vi "YokogawaGS200SweepAlexei.vi"() -> ()   [LabVIEW 2019]
panel:
  in  "INFINITE RUN status":bool caption="INFINITE RUN"
  in  "Set Time (s)":dbl=1.0 min=0.1 max=100.0 format="%.3f"
  out "Output Volt":dbl min=-10.0 max=10.0 format="%^.3e"
  in  "INFINITE RUN":bool
  in  "MODE:":enum32{"RAMP", "TRIANGLE"}(radio)=enum."TRIANGLE"
  in  "Step |Volt| (abs. value)":dbl=0.05 min=-1.0 max=1.0 format="%^.3e"
  in  "Delay per step OR ramp (s)":dbl=1.0 min=0.1 max=100.0 format="%.3f"
  in  "pause sweep":bool
  in  "Compliance Current":dbl format="%.3f"
  in  "Stop Volt":dbl=1.0 min=-10.0 max=10.0 format="%^.3e"
  in  "Start Volt":dbl min=-10.0 max=10.0 format="%^.3e"
  in  "Output Off":bool
  in  "Start Sweep":bool
  in  "Setup":bool
  in  "VISA resource name":refnum<visa-resource-name>
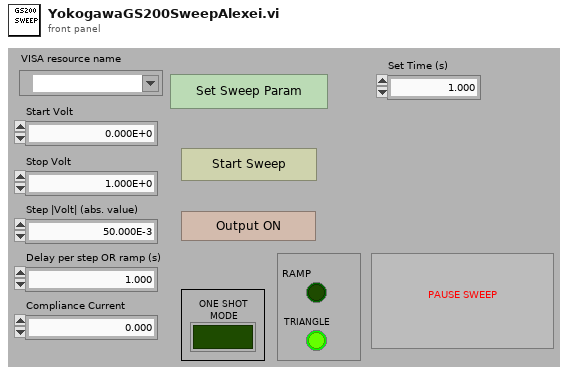
[diagram p1: front panel]
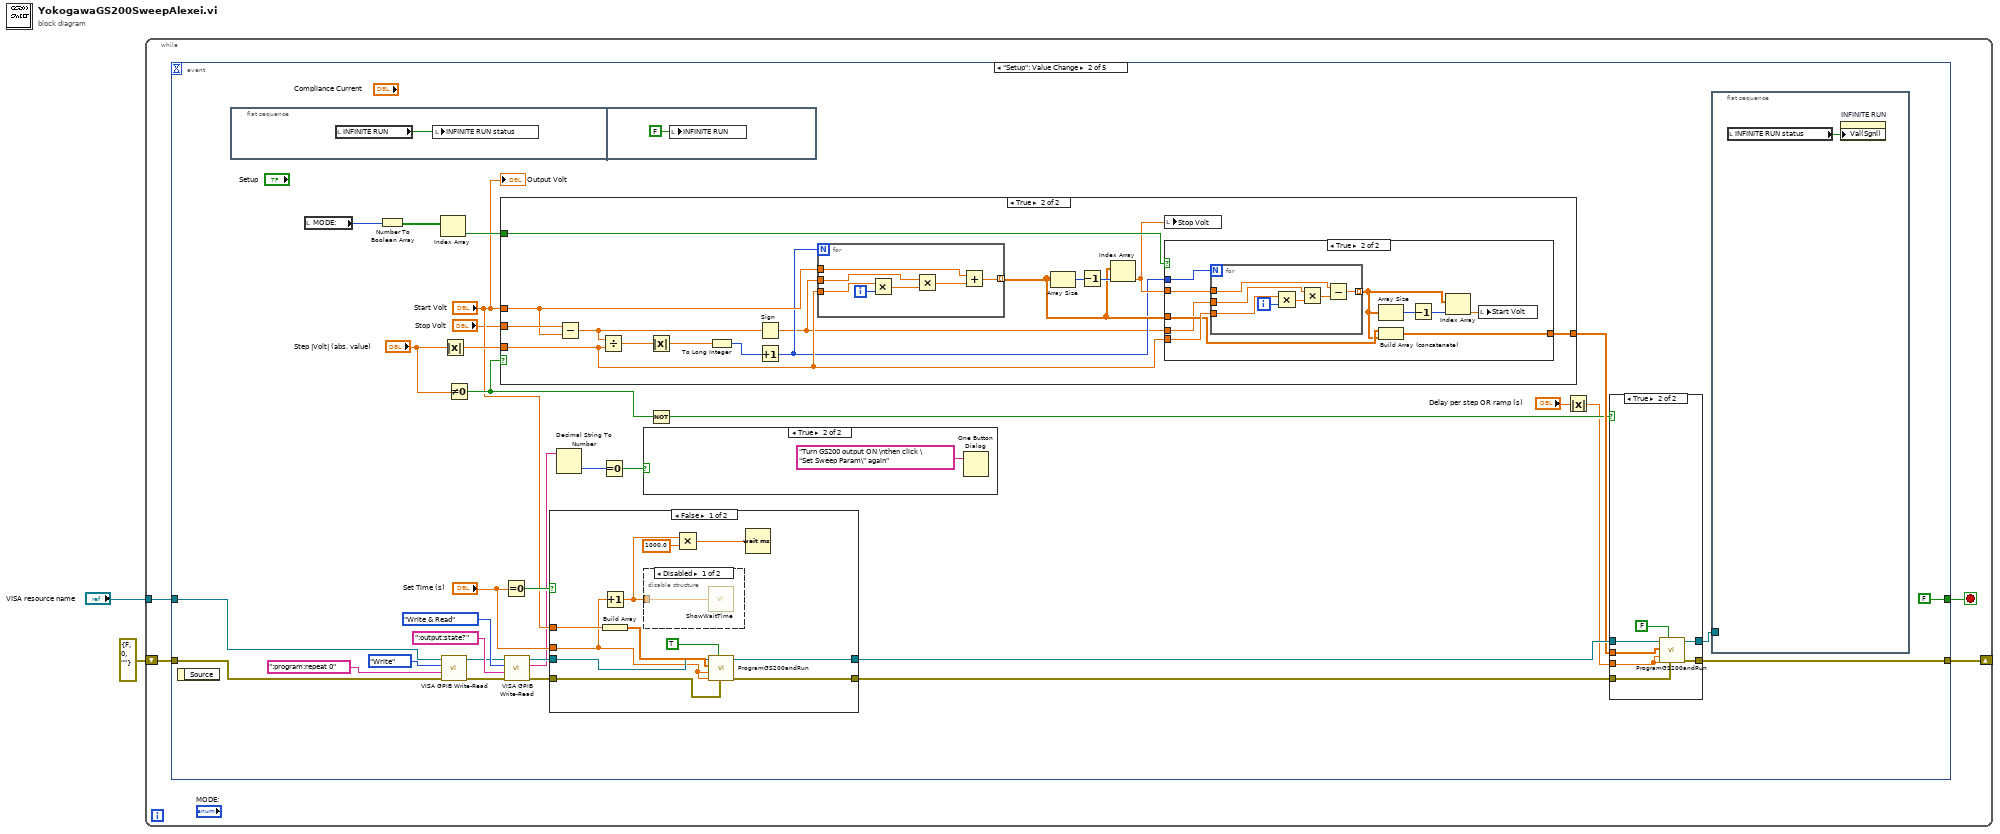
[diagram p0: block diagram]
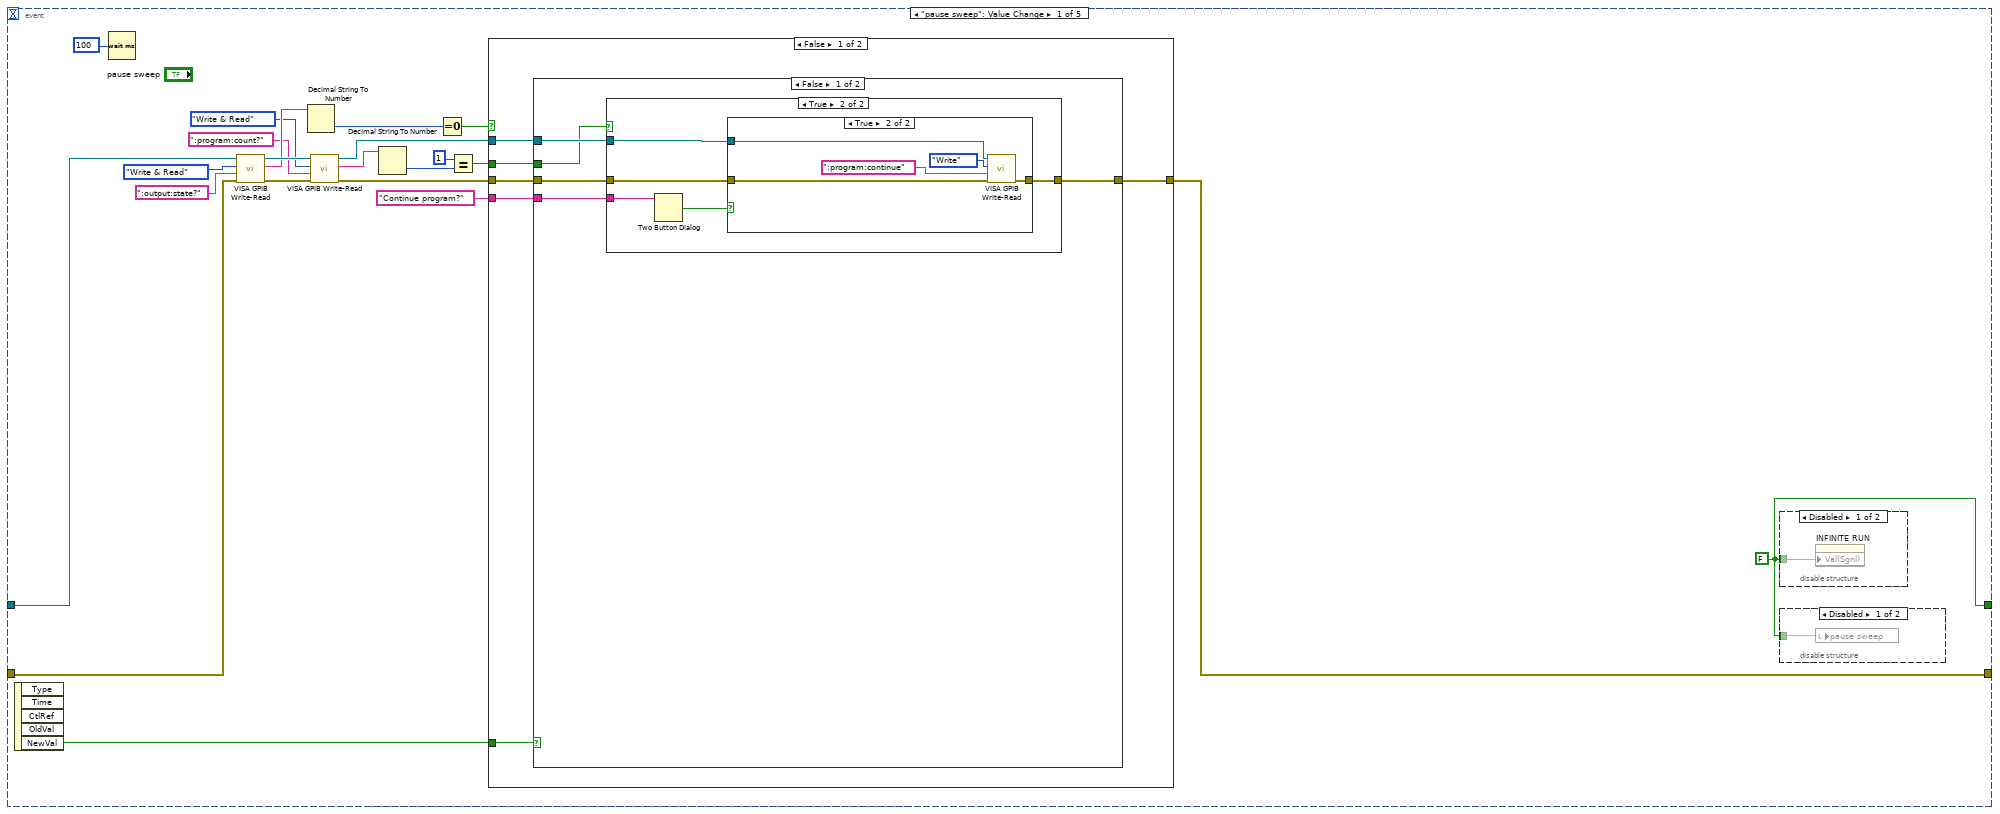
[diagram p2: hidden frame]
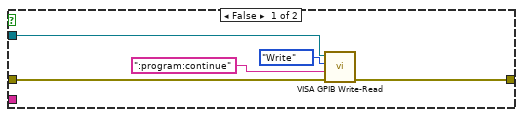
[diagram p4: hidden frame]
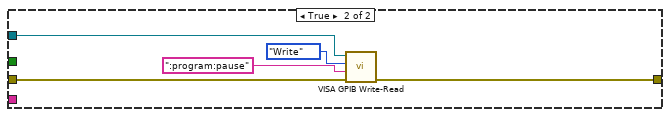
[diagram p6: hidden frame]
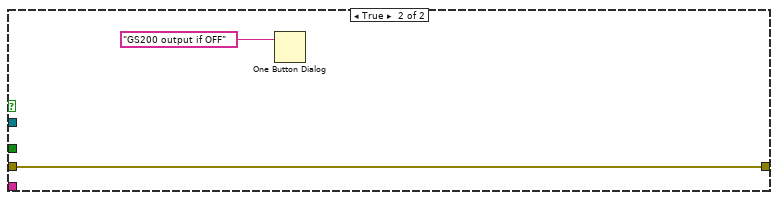
[diagram p7: hidden frame]
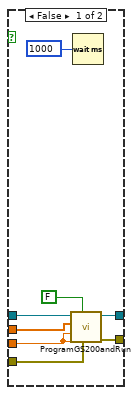
[diagram p9: hidden frame]
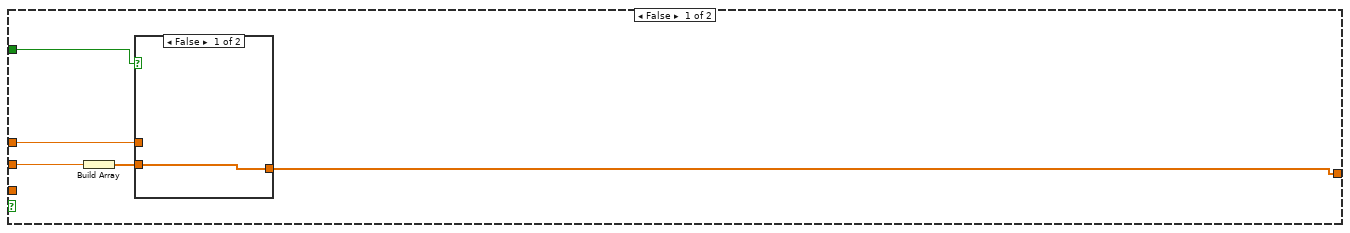
[diagram p11: hidden frame]
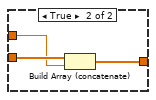
[diagram p12: hidden frame]
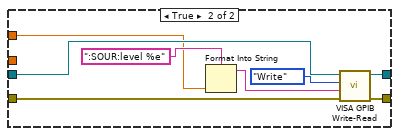
[diagram p15: hidden frame]
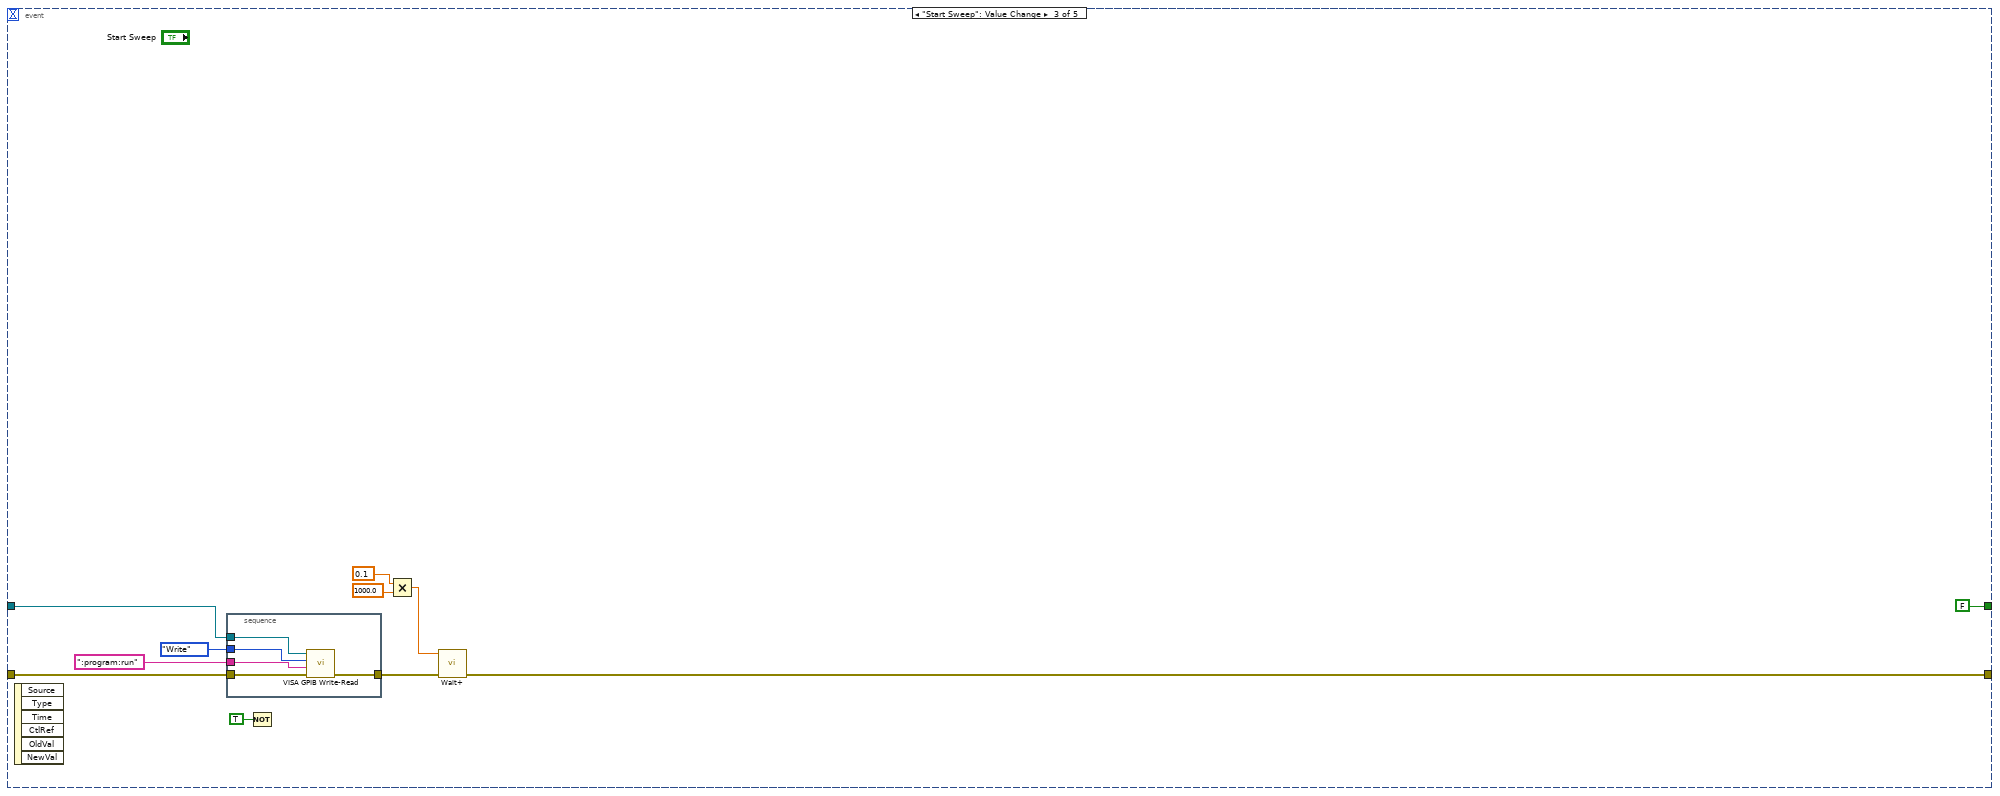
[diagram p16: hidden frame]
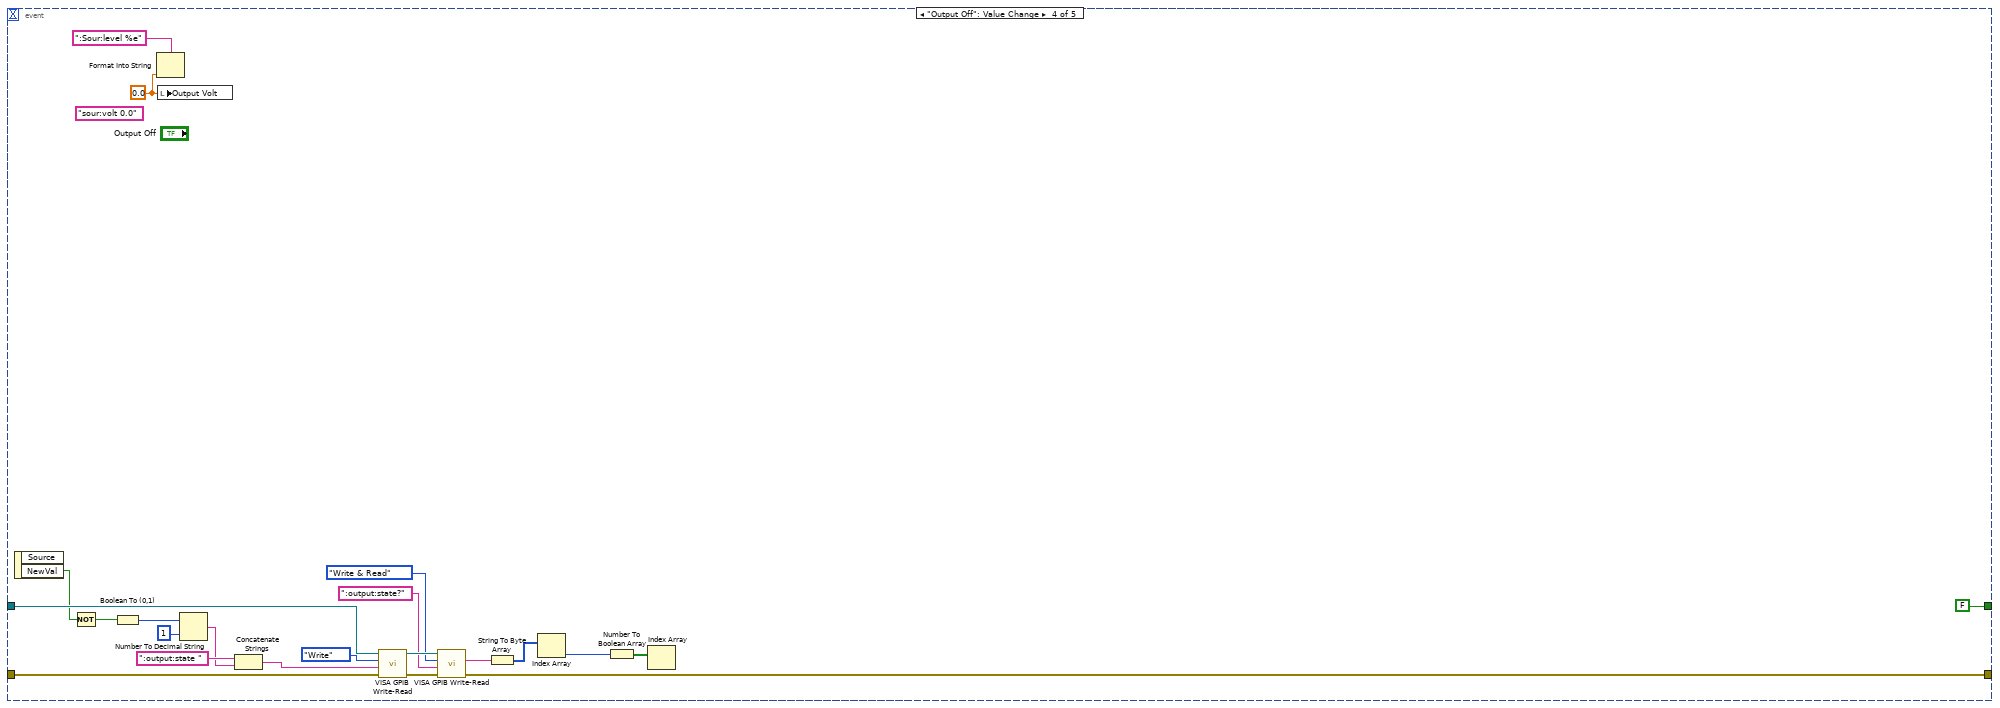
[diagram p17: hidden frame]
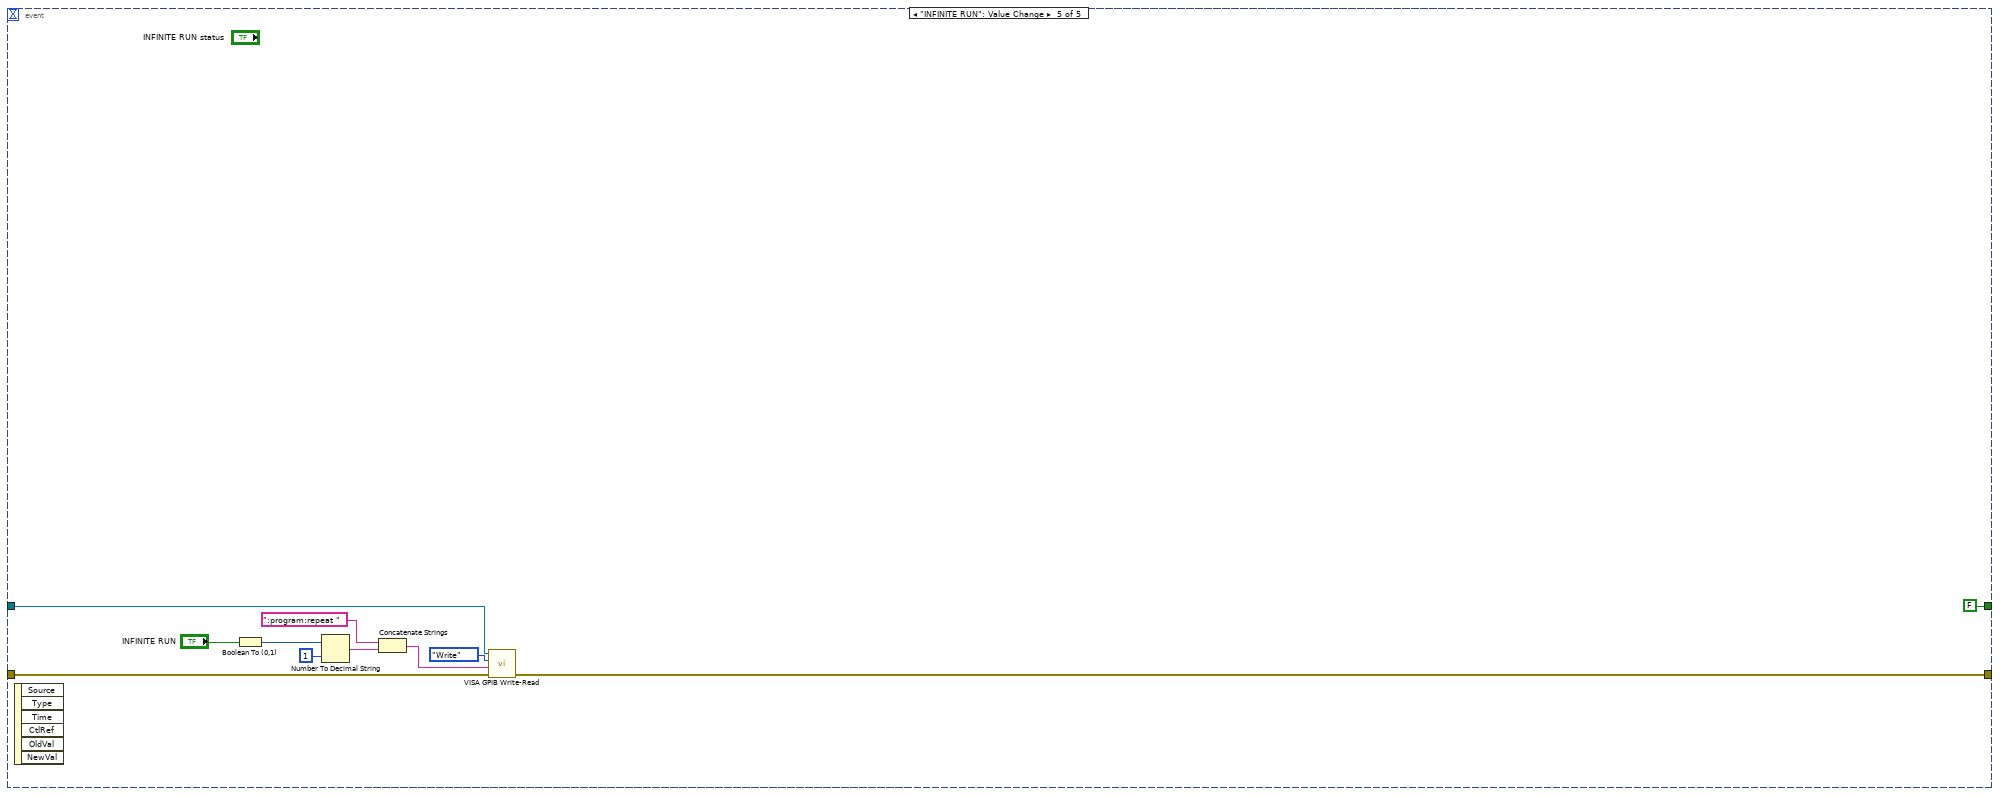
[diagram p18: hidden frame]
diagram:
  n1 = while {
    shift-right: [w5] -> _
    shift-left: errorcluster {"status"=FALSE, "code"=0, "source"=""} ("error out") -> [w4]
    tunnel: "VISA resource name" -> [w3]
    stop <- w6 stop-if-true
    n2 = event shown="[1] \"Setup\": Value Change" {
      selector: _ -> [_ _ _ _ _]
      dyn-events: _ -> [_ _ _ _ _]
      timeout: _ -> [_ _ _ _ _]
      tunnel: w3 -> [w26 w79 w195 w221 w227]
      tunnel: [w28 FALSE ("NewVal") FALSE ("NewVal") FALSE ("NewVal") FALSE ("NewVal")] -> w6
      tunnel: [w7 w67 w193 w220 w224] -> w5
      tunnel: w4 -> [w8 w66 w194 w219 w225]
      event "pause sweep": Value Change {
        w28 = FALSE ("stop")
        n3 = event-data() -> ("NewVal"=w27:bool)  [unwired: 1 in, 4 out]
        n4 = Wait (ms)(milliseconds to wait=u32 100) -> ()  [unwired: 1 out]
        n5 = call "VISA GPIB Write-Read.vi"("error in (no error)"=w8, "Command"=":output:state?" ("String to Write"), "Action"=enum16{"Write", "Read", "Write & Read"}."Write & Read", "VISA resource name"=w26) -> ("error out"=w10:errorcluster, "String Returned"=w19:string, "dup VISA Session"=w25:refnum<visa-resource-name>)  [unwired: 4 in, 1 out]
        n6 = Decimal String To Number(string=w19) -> (number=w20:i32)  [unwired: 2 in, 1 out]
        n7 = call "VISA GPIB Write-Read.vi"("error in (no error)"=w10, "Command"=":program:count?" ("String to Write"), "Action"=enum16{"Write", "Read", "Write & Read"}."Write & Read", "VISA resource name"=w25) -> ("error out"=w9:errorcluster, "String Returned"=w15:string, "dup VISA Session"=w16:refnum<visa-resource-name>)  [unwired: 4 in, 1 out]
        n8 = Decimal String To Number(string=w15) -> (number=w14:i32)  [unwired: 2 in, 1 out]
        n9 = Equal To 0?(x=w20) -> (x = 0?=w24:bool)
        n10 = Equal?(x=1, y=w14) -> (x = y?=w12:bool)
        n11 = case shown="False" w24 {
          tunnel: w16 -> [w35 _]
          tunnel: w27 -> [w34 _]
          tunnel: w12 -> [w33 _]
          tunnel: "Continue program?" ("message") -> [w32 _]
          tunnel: w9 -> [w31 w62]
          tunnel: [w30 w62] -> w7
          frame False {
            n12 = case shown="False" w34 {
              tunnel: w35 -> [w40 w59]
              tunnel: w33 -> [w39 _]
              tunnel: w32 -> [w38 _]
              tunnel: w31 -> [w37 w57]
              tunnel: [w36 w58] -> w30
              frame False {
                n13 = case shown="True" w39 {
                  tunnel: w40 -> [w43 w50]
                  tunnel: w38 -> [_ w48]
                  tunnel: w37 -> [w42 w47]
                  tunnel: [w41 w46] -> w36
                  frame False {
                    n14 = call "VISA GPIB Write-Read.vi"("error in (no error)"=w42, "Command"=":program:continue" ("String to Write"), "Action"=enum16{"Write", "Read", "Write & Read"}."Write", "VISA resource name"=w43) -> ("error out"=w41:errorcluster)  [unwired: 4 in, 3 out]
                  }
                  frame True {
                    n15 = Two Button Dialog(message=w48) -> (T button?=w49:bool)  [unwired: 2 in]
                    n16 = case shown="True" w49 {
                      tunnel: w50 -> [_ w54]
                      tunnel: w47 -> [w51 w53]
                      tunnel: [w51 w52] -> w46
                      frame False {
                      }
                      frame True {
                        n17 = call "VISA GPIB Write-Read.vi"("error in (no error)"=w53, "Command"=":program:continue" ("String to Write"), "Action"=enum16{"Write", "Read", "Write & Read"}."Write", "VISA resource name"=w54) -> ("error out"=w52:errorcluster)  [unwired: 4 in, 3 out]
                      }
                    }
                  }
                }
              }
              frame True {
                n18 = call "VISA GPIB Write-Read.vi"("error in (no error)"=w57, "Command"=":program:pause" ("String to Write"), "Action"=enum16{"Write", "Read", "Write & Read"}."Write", "VISA resource name"=w59) -> ("error out"=w58:errorcluster)  [unwired: 4 in, 3 out]
              }
            }
          }
          frame True {
            n19 = One Button Dialog(message="GS200 output if OFF") -> ()  [unwired: 1 in, 1 out]
          }
        }
        n20 = disable-structure shown="Disabled" {
          disable-tunnel: w28 -> [w29 _]
          frame Disabled {
            n21 = property on="INFINITE RUN" class="Bool (strict)"("Val(Sgnl)"=w29) -> ()  [unwired: 2 in, 2 out]
          }
          frame Enabled {
          }
        }
        n22 = disable-structure shown="Disabled" {
          disable-tunnel: w28 -> [w64 _]
          frame Disabled {
            n23 = local write "pause sweep"(w64) -> ()
          }
          frame Enabled {
          }
        }
      }
      event "Setup": Value Change {
        n24 = event-data() -> ()  [unwired: 1 in, 1 out]
        n25 = flat-sequence {
          frame #0 {
            n26 = local read "INFINITE RUN"() -> (w114:bool)
            n27 = local write "INFINITE RUN status"(w114) -> ()
          }
          frame #1 {
            n28 = local write "INFINITE RUN"(FALSE ("INFINITE RUN")) -> ()
          }
        }
        n29 = local read "MODE:"() -> (w89:enum32{"RAMP", "TRIANGLE"})
        n30 = Number To Boolean Array(number=w89) -> (Boolean array=w93:bool[])
        n31 = Index Array(array=w93) -> (element=w90:bool)  [unwired: 1 in]
        n32 = call "VISA GPIB Write-Read.vi"("error in (no error)"=w66, "Command"=":program:repeat 0", "Action"=enum16{"Write", "Read", "Write & Read"}."Write", "VISA resource name"=w79) -> ("error out"=w73:errorcluster, "dup VISA Session"=w75:refnum<visa-resource-name>)  [unwired: 4 in, 2 out]
        n33 = Absolute Value(x="Step |Volt| (abs. value)") -> (abs(x)=w86:dbl)
        n34 = Not Equal To 0?(x="Step |Volt| (abs. value)") -> (x != 0?=w88:bool)
        n35 = case shown="True" w88 {
          tunnel: w86 -> [_ w130]
          tunnel: "Stop Volt" -> [w120 w137]
          tunnel: "Start Volt" -> [w116 w136]
          tunnel: [w117 w131] -> w91
          tunnel: w90 -> [w119 w133]
          frame False {
            n36 = Build Array(w120) -> (w118:dbl[])
            n37 = case shown="False" w119 {
              tunnel: w118 -> [w121 w124]
              tunnel: [w121 w122] -> w117
              tunnel: w116 -> [_ w123]
              frame False {
              }
              frame True {
                n38 = Build Array (concatenate)(w124, w123) -> (w122:dbl[])
              }
            }
          }
          frame True {
            n39 = Subtract(x=w137, y=w136) -> (x-y=w127:dbl)
            n40 = Divide(x=w127, y=w130) -> (x/y=w139:dbl)
            n41 = Absolute Value(x=w139) -> (abs(x)=w125:dbl)
            n42 = To Long Integer(number=w125) -> (32bit integer=w138:i32)
            n43 = Sign(1:w127) -> (0:w126:dbl)
            n44 = Increment(x=w138) -> (x+1=w128:i32)
            n45 = for {
              N: w128 -> [_]
              tunnel: w136 -> [w161]
              tunnel: w130 -> [w162]
              tunnel: [w160] -> w132 mode=indexing
              tunnel: w126 -> [w158]
              i -> [w163]
              n46 = Multiply(x=w162, y=w163) -> (x*y=w164:dbl)
              n47 = Multiply(x=w158, y=w164) -> (x*y=w159:dbl)
              n48 = Add(x=w161, y=w159) -> (x+y=w160:dbl)
            }
            n49 = Array Size(array=w132) -> (size(s)=w135:i32)
            n50 = Decrement(x=w135) -> (x-1=w134:i32)
            n51 = Index Array(array=w132, index=w134) -> (element=w129:dbl)
            n52 = local write "Stop Volt"(w129) -> ()
            n53 = case shown="True" w133 {
              tunnel: w132 -> [w140 w147]
              tunnel: [w140 w143] -> w131
              tunnel: w130 -> [_ w150]
              tunnel: w129 -> [_ w149]
              tunnel: w128 -> [_ w148]
              tunnel: w126 -> [_ w141]
              frame False {
              }
              frame True {
                n54 = for {
                  N: w148 -> [_]
                  tunnel: w149 -> [w154]
                  tunnel: w150 -> [w155]
                  tunnel: [w153] -> w142 mode=indexing
                  tunnel: w141 -> [w151]
                  i -> [w156]
                  n55 = Multiply(x=w155, y=w156) -> (x*y=w157:dbl)
                  n56 = Multiply(x=w151, y=w157) -> (x*y=w152:dbl)
                  n57 = Subtract(x=w154, y=w152) -> (x-y=w153:dbl)
                }
                n58 = Array Size(array=w142) -> (size(s)=w146:i32)
                n59 = Build Array (concatenate)(w147, w142) -> (w143:dbl[])
                n60 = Decrement(x=w146) -> (x-1=w145:i32)
                n61 = Index Array(array=w142, index=w145) -> (element=w144:dbl)
                n62 = local write "Start Volt"(w144) -> ()
              }
            }
          }
        }
        n63 = Equal To 0?(x="Set Time (s)") -> (x = 0?=w95:bool)
        n64 = call "VISA GPIB Write-Read.vi"("error in (no error)"=w73, "Command"=":output:state?" ("String to Write"), "Action"=enum16{"Write", "Read", "Write & Read"}."Write & Read", "VISA resource name"=w75) -> ("error out"=w65:errorcluster, "String Returned"=w70:string, "dup VISA Session"=w74:refnum<visa-resource-name>)  [unwired: 4 in, 1 out]
        n65 = case shown="False" w95 {
          tunnel: w65 -> [w167 w181]
          tunnel: [w175 w180] -> w68
          tunnel: w74 -> [w169 w183]
          tunnel: "Set Time (s)" -> [w166 _]
          tunnel: "Start Volt" -> [w171 w178]
          tunnel: [w168 w177] -> w92
          frame False {
            n66 = Increment(x=w166) -> (x+1=w165:dbl)
            n67 = Build Array(w171) -> (w172:dbl[])
            n68 = disable-structure shown="Disabled" {
              disable-tunnel: w165 -> [w176 _]
              frame Disabled {
                n69 = call "ShowWaitTime.vi"("Delay (sec)"=w176) -> ()  [unwired: 1 out]
              }
              frame Enabled {
              }
            }
            n70 = Multiply(x=w165, y=1000.0) -> (x*y=w170:dbl)
            n71 = call "ProgramGS200andRun.vi"("error in"=w167, "Run program?"=TRUE, "Interval input"=w166, "Slope Input"=w166, "Voltage array"=w172, "VISA resource name"=w169) -> ("error out"=w175:errorcluster, "VISA resource name out"=w168:refnum<visa-resource-name>)  [unwired: 3 in]
            n72 = Wait (ms)(milliseconds to wait=w170) -> ()  [unwired: 1 out]
          }
          frame True {
            n73 = Format Into String(format string=":SOUR:level %e", w178) -> (resulting string=w182:string)  [unwired: 2 in, 1 out]
            n74 = call "VISA GPIB Write-Read.vi"("error in (no error)"=w181, "Command"=w182, "Action"=enum16{"Write", "Read", "Write & Read"}."Write", "VISA resource name"=w183) -> ("error out"=w180:errorcluster, "dup VISA Session"=w177:refnum<visa-resource-name>)  [unwired: 4 in, 2 out]
          }
        }
        n75 = Decimal String To Number(string=w70) -> (number=w72:i32)  [unwired: 2 in, 1 out]
        n76 = Equal To 0?(x=w72) -> (x = 0?=w71:bool)
        n77 = case shown="True" w71 {
          frame False {
          }
          frame True {
            n78 = One Button Dialog(message="Turn GS200 output ON \nthen click \"Set Sweep Param\" again") -> ()  [unwired: 1 in, 1 out]
          }
        }
        n79 = Not(x=w88) -> (.not. x?=w87:bool)
        n80 = Absolute Value(x="Delay per step OR ramp (s)") -> (abs(x)=w84:dbl)
        n81 = case shown="True" w87 {
          tunnel: w92 -> [w104 w112]
          tunnel: w91 -> [w103 w111]
          tunnel: w84 -> [w101 w109]
          tunnel: [w100 w107] -> w69
          tunnel: w68 -> [w99 w108]
          tunnel: [w98 w106] -> w67
          frame False {
            n82 = call "ProgramGS200andRun.vi"("error in"=w99, "Run program?"=FALSE, "Interval input"=w101, "Slope Input"=w101, "Voltage array"=w103, "VISA resource name"=w104) -> ("error out"=w98:errorcluster, "VISA resource name out"=w100:refnum<visa-resource-name>)  [unwired: 3 in]
            n83 = Wait (ms)(milliseconds to wait=u32 1000) -> ()  [unwired: 1 out]
          }
          frame True {
            n84 = call "ProgramGS200andRun.vi"("error in"=w108, "Run program?"=FALSE, "Interval input"=w109, "Slope Input"=w109, "Voltage array"=w111, "VISA resource name"=w112) -> ("error out"=w106:errorcluster, "VISA resource name out"=w107:refnum<visa-resource-name>)  [unwired: 3 in]
          }
        }
        n85 = flat-sequence {
          tunnel: w69 -> [_]
          frame #0 {
            n86 = local read "INFINITE RUN status"() -> (w97:bool)
            n87 = property on="INFINITE RUN" class="Bool (strict)"("Val(Sgnl)"=w97) -> ()  [unwired: 2 in, 2 out]
          }
        }
        "Output Volt" <- "Start Volt"
      }
      event "Start Sweep": Value Change {
        n88 = event-data() -> ()  [unwired: 1 in, 6 out]
        n89 = stacked-sequence {
          tunnel: w195 -> [w200]
          tunnel: w194 -> [w199]
          tunnel: [w196] -> w191
          tunnel: enum16{"Write", "Read", "Write & Read"}."Write" ("Action") -> [w198]
          tunnel: ":program:run" -> [w197]
          frame #0 {
            n90 = call "VISA GPIB Write-Read.vi"("error in (no error)"=w199, "Command"=w197, "Action"=w198, "VISA resource name"=w200) -> ("error out"=w196:errorcluster)  [unwired: 4 in, 3 out]
          }
        }
        n91 = Not(x=TRUE) -> ()  [unwired: 1 out]
        n92 = Multiply(x=0.1, y=1000.0) -> (x*y=w185:dbl)
        n93 = call "Wait+.vi"("Error In"=w191, "milliseconds to wait"=w185) -> ("Error Out"=w193:errorcluster)  [unwired: 4 in, 1 out]
      }
      event "Output Off": Value Change {
        w217 = 0.0 ("Output Volt 2")
        (unwired) "sour:volt 0.0"
        n94 = event-data() -> ("NewVal"=w212:bool)  [unwired: 1 in, 1 out]
        n95 = Not(x=w212) -> (.not. x?=w211:bool)
        n96 = Boolean To (0,1)(Boolean=w211) -> (0, 1=w215:i16)
        n97 = Format Into String(format string=":Sour:level %e", w217) -> ()  [unwired: 2 in, 2 out]
        n98 = local write "Output Volt"(w217) -> ()
        n99 = Number To Decimal String(number=w215, width (-)=i16 1) -> (decimal integer string=w213:string)
        n100 = Concatenate Strings(":output:state " ("String to Write"), w213) -> (w207:string)
        n101 = call "VISA GPIB Write-Read.vi"("error in (no error)"=w219, "Command"=w207, "Action"=enum16{"Write", "Read", "Write & Read"}."Write", "VISA resource name"=w221) -> ("error out"=w210:errorcluster, "dup VISA Session"=w209:refnum<visa-resource-name>)  [unwired: 4 in, 2 out]
        n102 = call "VISA GPIB Write-Read.vi"("error in (no error)"=w210, "Command"=":output:state?" ("String to Write"), "Action"=enum16{"Write", "Read", "Write & Read"}."Write & Read", "VISA resource name"=w209) -> ("error out"=w220:errorcluster, "String Returned"=w204:string)  [unwired: 4 in, 2 out]
        n103 = String To Byte Array(string=w204) -> (unsigned byte array=w203:u8[])
        n104 = Index Array(array=w203) -> (element=w202:u8)  [unwired: 1 in]
        n105 = Number To Boolean Array(number=w202) -> (Boolean array=w201:bool[])
        n106 = Index Array(array=w201) -> ()  [unwired: 1 in, 1 out]
      }
      event "INFINITE RUN": Value Change {
        n107 = event-data() -> ()  [unwired: 1 in, 6 out]
        n108 = Boolean To (0,1)(Boolean="INFINITE RUN") -> (0, 1=w232:i16)
        n109 = Number To Decimal String(number=w232, width (-)=i16 1) -> (decimal integer string=w230:string)
        n110 = Concatenate Strings(":program:repeat ", w230) -> (w228:string)
        n111 = call "VISA GPIB Write-Read.vi"("error in (no error)"=w225, "Command"=w228, "Action"=enum16{"Write", "Read", "Write & Read"}."Write", "VISA resource name"=w227) -> ("error out"=w224:errorcluster)  [unwired: 4 in, 3 out]
      }
    }
  }
